vi "Ex2_AverageValue.vi"() -> ()   [LabVIEW 2024]
panel:
  out "Result":dbl
  in  "Student 3":dbl
  in  "Student 2":dbl
  in  "Student 1":dbl
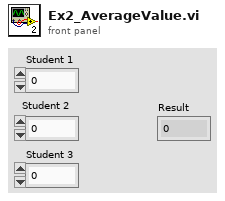
[diagram p1: front panel]
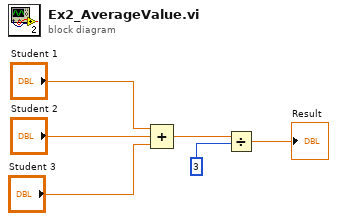
[diagram p0: block diagram]
diagram:
  n1 = Compound Arithmetic op=ADD("Student 1", "Student 2", "Student 3") -> (w3:dbl)
  n2 = Divide(x=w3, y=3) -> (x/y=→"Result":dbl)
